vi "Get Object from String.vi"(8 "error in":errorcluster, 9 "Sub-Index":string, 10 "Index":string, 11 "Sorted Object Dictionary in":refnum<class "Sorted Object Dictionary.lvclass">) -> (0 "error out":errorcluster, 1 "OD Entry":refnum<class "OD Entry.lvclass">, 2 "Found?":bool, 3 "Sorted Object Dictionary out":refnum<class "Sorted Object Dictionary.lvclass">)   [LabVIEW 2024, in "EDS.lvlib" / "Sorted Object Dictionary.lvclass"]
uses:
  Sorted Object Dictionary.lvclass
  OD Entry/OD Entry.lvclass
  Sorted Object Dictionary.lvclass/Sorted Object Dictionary.ctl
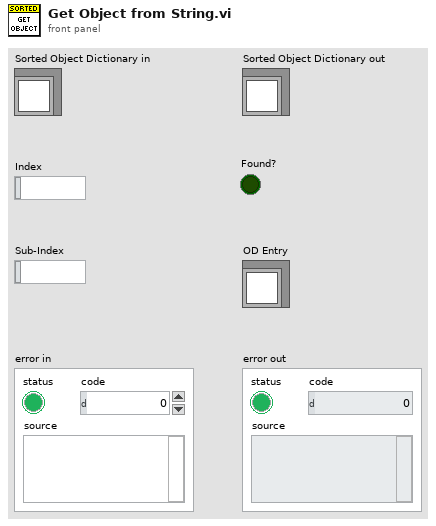
[diagram p1: front panel]
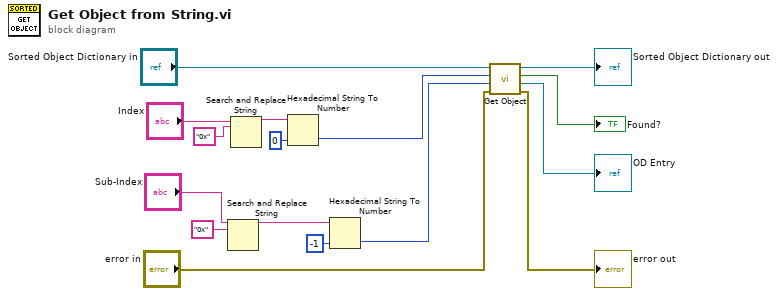
[diagram p0: block diagram]
diagram:
  n1 = Search and Replace String(input string="Sub-Index", search string="0x") -> (result string=w9:string)  [unwired: 6 in, 3 out]
  n2 = Search and Replace String(input string="Index", search string="0x") -> (result string=w7:string)  [unwired: 6 in, 3 out]
  n3 = Hexadecimal String To Number(string=w7, default (0uL)=u16 0 ("default (0 U32)")) -> (number=w5:u16)  [unwired: 1 in, 1 out]
  n4 = Hexadecimal String To Number(string=w9, default (0uL)=i16 -1 ("default (0 U32)")) -> (number=w8:i16)  [unwired: 1 in, 1 out]
  n5 = call "Get Object.vi"("error in"="error in", "Sub-Index"=w8, "Index"=w5, "Sorted Object Dictionary in"="Sorted Object Dictionary in") -> ("error out"=→"error out":errorcluster, "OD Entry"=→"OD Entry":refnum<class "OD Entry.lvclass">, "Found?"=→"Found?":bool, "Sorted Object Dictionary out"=→"Sorted Object Dictionary out":refnum<class "Sorted Object Dictionary.lvclass">)  [unwired: 4 in]
